vi "ma_SML Spectrum (real input).vi"(2 "FFT Size":i32, 3 "window":u16(ring) items=["Rectangle"=0, "Hanning"=1, "Hamming"=2, "Blackman-Harris"=3, "Exact Blackman"=4, "Blackman"=5, "Flat Top"=6, "4 Term B-Harris "=7, "7 Term B-Harris"=8, "Low Sidelobe"=9, "Blackman Nuttall"=11, "Triangle"=30, "Bartlett-Hanning"=31, "Bohman"=32, "Parzen"=33, "Welch"=34, "Kaiser"=60, "Dolph-Chebyshev"=61, "Gaussian"=62], 4 "x[V]":dbl[](array[numeric]) format="%.2f") -> (0 "spectral info":T1 {"window" items=["Rectangle"=0, "Hanning"=1, "Hamming"=2, "Blackman-Harris"=3, "Exact Blackman"=4, "Blackman"=5, "Flat Top"=6, "4 Term B-Harris "=7, "7 Term B-Harris"=8, "Low Sidelobe"=9, "Blackman Nuttall"=11, "Triangle"=30, "Bartlett-Hanning"=31, "Bohman"=32, "Parzen"=33, "Welch"=34, "Kaiser"=60, "Dolph-Chebyshev"=61, "Gaussian"=62]}, 1 "FFT{x} [Vrms]":cdb[](array[numeric]) format="%.2f")   [LabVIEW 2020, in "NI_MAPro.lvlib"]
uses:
  NI_MAPro.lvlib
  ma_sml_Spectral Info.ctl
  NI_AALPro.lvlib
panel:
  # "Real signal's Windowed, normalized SSB spectrum"
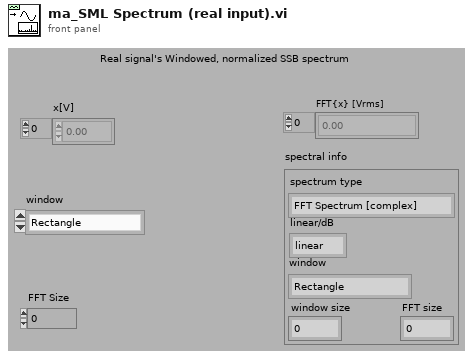
[diagram p1: front panel]
types:
  T1 = typedef "NI_MAPro.lvlib/ma_sml_Spectral Info.ctl" = cluster{"spectrum type":enum16{"FFT Spectrum [complex]", "Amplitude [Magnitude]", "Power [Magnitude^2]", "Cross Spectrum [complex]", "Frequency Response [Complex]"}, "linear/dB":enum16{"linear", "dB"}, "window":u16, "window size":i32, "FFT size":i32}
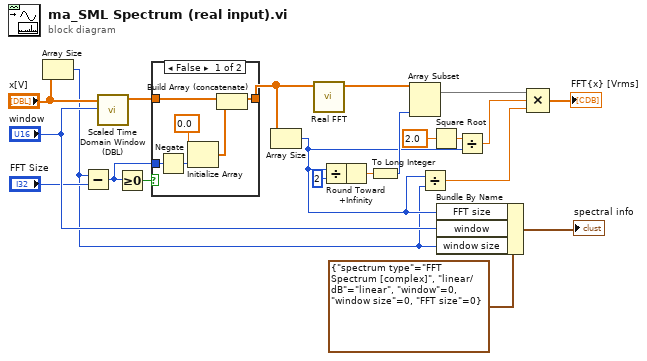
[diagram p0: block diagram]
diagram:
  n1 = Array Size(array="x[V]") -> (size(s)=w3:i32)
  n2 = Subtract(x=w3, y="FFT Size") -> (x-y=w12:i32)
  n3 = call "Scaled Time Domain Window (DBL).vi"("window"="window", "X"="x[V]") -> ("Windowed X"=w13:dbl[])  [unwired: 7 in, 2 out]
  n4 = Greater Or Equal To 0?(x=w12) -> (x >= 0?=w11:bool)
  n5 = case shown="False" w11 {
    tunnel: w13 -> [w25 w29]
    tunnel: [w26 w29] -> w8
    tunnel: w12 -> [w27 _]
    frame False {
      n6 = Negate(x=w27) -> (-x=w23:i32)
      n7 = Initialize Array(0.0 ("Element Data"), w23) -> (w24:dbl[])
      n8 = Build Array (concatenate)(w25, w24) -> (w26:dbl[])
    }
    frame True {
    }
  }
  n9 = Array Size(array=w8) -> (size(s)=w4:i32)
  n10 = call "Real FFT.vi"("X"=w8) -> ("FFT {X}"=w22:cdb[])  [unwired: 9 in, 1 out]
  n11 = Divide(x=w4, y=2) -> (x/y=w16:dbl)
  n12 = Round Toward +Infinity(x=w16) -> (ceil(x): smallest int >= x=w19:dbl)
  n13 = To Long Integer(number=w19) -> (32bit integer=w18:i32)
  n14 = Array Subset(array=w22, length=w18) -> (w17:cdb[])  [unwired: 1 in]
  n15 = Divide(x=w4, y=w3) -> (x/y=w2:dbl)
  n16 = Square Root(x=2.0 ("y")) -> (sqrt(x)=w5:dbl)
  n17 = Bundle By Name(cluster=T1 {"spectrum type"=enum."FFT Spectrum [complex]", "linear/dB"=enum."linear", "window"=0, "window size"=0, "FFT size"=0} ("spectral info"), "FFT size"=w4, "window"="window", "window size"=w3) -> (→"spectral info":T1)
  n18 = Divide(x=w5, y=w4) -> (x/y=w15:dbl)
  n19 = Compound Arithmetic op=MULTIPLY(w17, w15, w2) -> (→"FFT{x} [Vrms]":cdb[])
